vi "Write Displacement Sensor Serial.vi"(10 "SerialProtocols.lvlib:SerialReal.lvclass":refnum<class "SerialReal.lvclass">, 11 "Model in":refnum<class "Model.lvclass">) -> (3 "Model out":refnum<class "Model.lvclass">)   [LabVIEW 2016, in "Model.lvclass"]
uses:
  Model.lvclass
  Common_SerialProtocols/SerialProtocol/SerialReal/SerialReal.lvclass
  Model.lvclass/Model.ctl
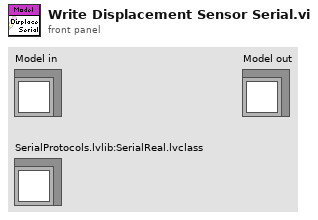
[diagram p1: front panel]
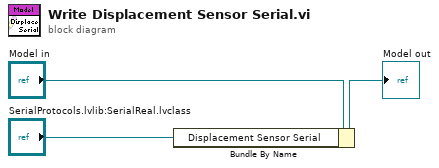
[diagram p0: block diagram]
diagram:
  n1 = Bundle By Name(cluster="Model in", "Displacement Sensor Serial"="SerialProtocols.lvlib:SerialReal.lvclass") -> (→"Model out":refnum<class "Model.lvclass">)
